vi "Set State_Measure iVIO and Resistance.vi"(0 "Semiconductor Module Context":T3, 1 "script name":string, 5 "Pins":string[](array[string])=["VDD"], 7 "Power_Pins":string[](array[string]), 9 "Published Data Ids":string[](array[string]), 11 "error in (no error)":errorcluster, 12 "SMU Settings":T2={"Level"=0.01, "Level Range"=0.1, "Limit"=1.0, "Limit Range"=6.0, "Sense"=1009} {"Sense" items=["Local"=1008, "Remote"=1009]}) -> (15 "error out":errorcluster)   [LabVIEW 2013]
uses:
  <vilib>/NI_TestStand_SemiconductorModule/NI_TestStand_Semiconductor_Module.lvlibp/PinMap/General/SemiconductorModuleContext.ctl
  <instrlib>/niDCPower/nidcpower.llb/niDCPower Sense.ctl
  <instrlib>/niHSDIO/niHSDIO.llb/niHSDIO_ctl Trigger Script - trigID Values (Ring).ctl
  <vilib>/NI_TestStand_SemiconductorModule/NI_TestStand_Semiconductor_Module.lvlibp/PinMap/DC Power/PinsToNIDCPowerSessions.vi
  <vilib>/NI_TestStand_SemiconductorModule/NI_TestStand_Semiconductor_Module.lvlibp/PinMap/General/Publish/PublishDataDouble2D.vi
  <vilib>/NI_TestStand_SemiconductorModule/NI_TestStand_Semiconductor_Module.lvlibp
panel:
  out "current measurements":dbl[][](array[numeric])
  out "R Array":dbl[][](array[numeric]) format="%#_6p"
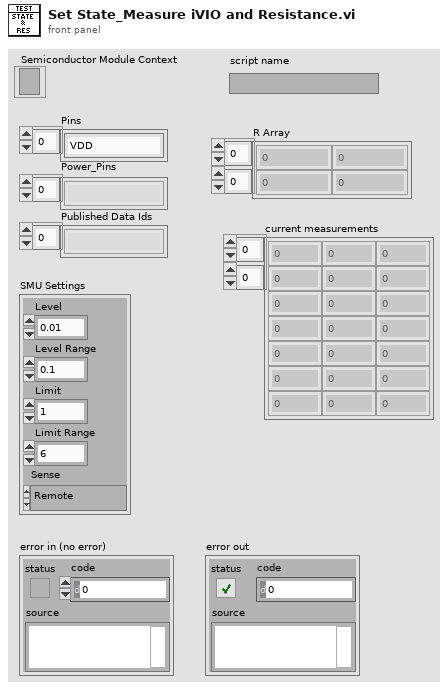
[diagram p1: front panel]
types:
  T1 = typedef "niDCPower Sense.ctl" = i32
  T2 = cluster{"Level":dbl, "Level Range":dbl, "Limit":dbl, "Limit Range":dbl, "Sense":T1}
  T3 = typedef "NI_TestStand_Semiconductor_Module.lvlibp/SemiconductorModuleContext.ctl" = refnum<k7>
  T4 = typedef "niHSDIO_ctl Trigger Script - trigID Values (Ring).ctl" = string
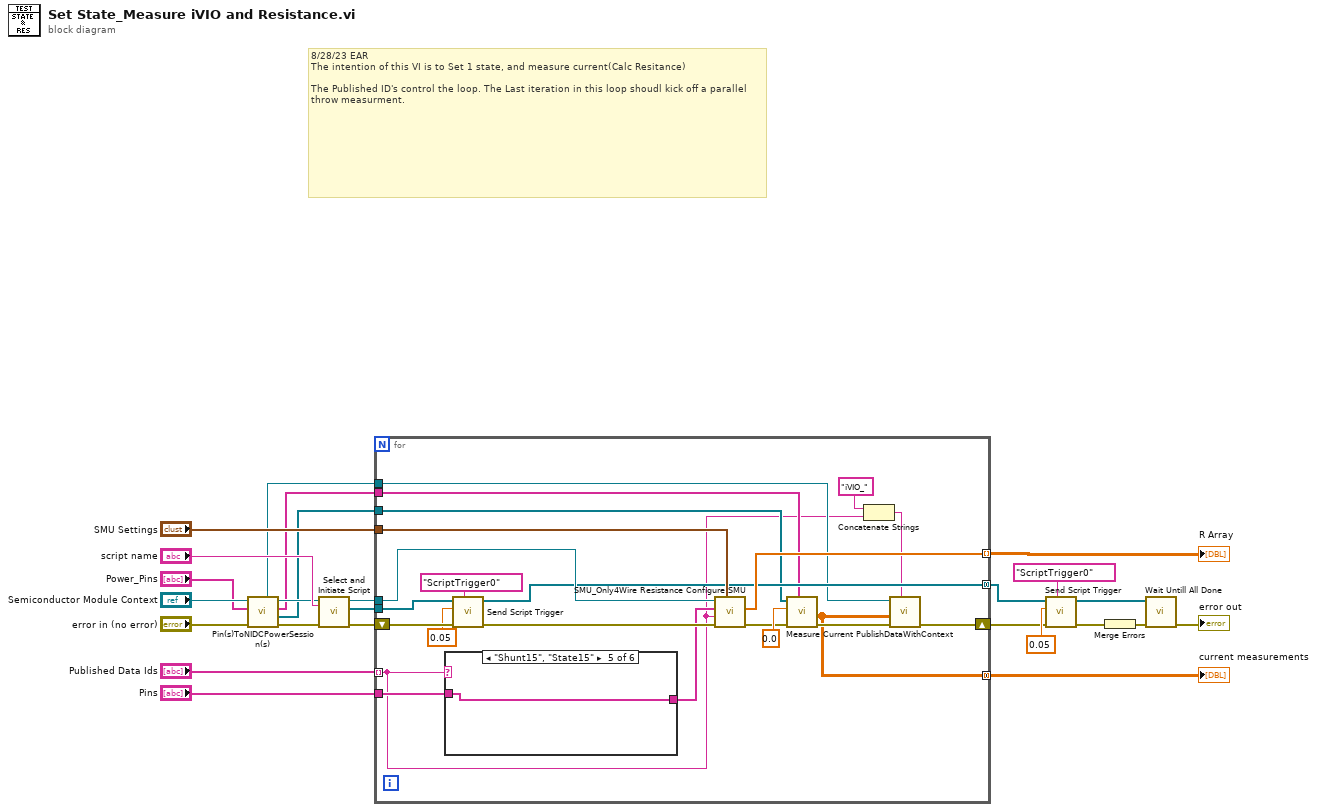
[diagram p0: block diagram]
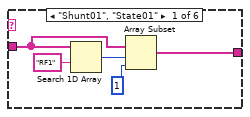
[diagram p2: hidden frame]
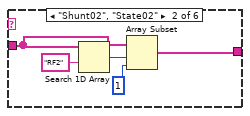
[diagram p3: hidden frame]
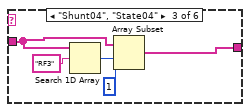
[diagram p4: hidden frame]
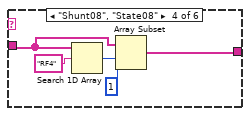
[diagram p5: hidden frame]
diagram:
  # "8/28/23 EAR\nThe intention of this VI is to Set 1 state, and measure current(Calc Resitance)\n\nThe Published ID's control the loop. The Last iteration in this loop shoudl kick off a parallel throw measurment."
  n1 = call-poly <vilib>:"Pin(s)ToNIDCPowerSession(s).vi"("error in (no error)"="error in (no error)", "Pins"="Power_Pins", "Semiconductor Module Context"="Semiconductor Module Context") -> ("error out"=w10:errorcluster, "Instrument Sessions"=w5:refnum<k15>[], "Channel Lists"=w4:string[], "Semiconductor Module Context Out"=w7:T3, "Pin Query Context"=w2:refnum<class "MultiplePinMultipleSessionQueryContext.lvclass">)  [unwired: 4 in]
  n2 = call "Select and Initiate Script.vi"("error in (no error)"=w10, "script name"="script name", "Semiconductor Module Context"=w7) -> ("error out"=w25:errorcluster, "HSDIO GEN Sessions Out"=w24:refnum<k15>[], "Semiconductor Module Context Out"=w21:T3)  [unwired: 6 in]
  n3 = for {
    tunnel: w24 -> [w46]
    tunnel: "SMU Settings" -> [w45]
    tunnel: w21 -> [w44]
    tunnel: "Published Data Ids" -> [w28] mode=indexing
    tunnel: "Pins" -> [w40]
    tunnel: [w41] -> w18 mode=indexing
    tunnel: [w38] -> w13 mode=concatenating
    shift-right: [w31] -> w3
    shift-left: w25 -> [w47]
    tunnel: w5 -> [w33]
    tunnel: w4 -> [w34]
    tunnel: w2 -> [w30]
    tunnel: [w29] -> w1 mode=concatenating
    n4 = case shown="\"Shunt15\", \"State15\"" w28 {
      tunnel: w40 -> [w51 w54 w61 w63 w68 w69]
      tunnel: [w50 w53 w60 w64 w68 w69] -> w39
      frame "Shunt01", "State01" {
        n5 = Search 1D Array(1D array=w51, element="RF1") -> (index of element=w49:i32)  [unwired: 1 in]
        n6 = Array Subset(array=w51, index=w49, length=1) -> (w50:string[])
      }
      frame "Shunt02", "State02" {
        n7 = Search 1D Array(1D array=w54, element="RF2") -> (index of element=w56:i32)  [unwired: 1 in]
        n8 = Array Subset(array=w54, index=w56, length=1) -> (w53:string[])
      }
      frame "Shunt04", "State04" {
        n9 = Search 1D Array(1D array=w61, element="RF3") -> (index of element=w59:i32)  [unwired: 1 in]
        n10 = Array Subset(array=w61, index=w59, length=1) -> (w60:string[])
      }
      frame "Shunt08", "State08" {
        n11 = Search 1D Array(1D array=w63, element="RF4") -> (index of element=w66:i32)  [unwired: 1 in]
        n12 = Array Subset(array=w63, index=w66, length=1) -> (w64:string[])
      }
      frame "Shunt15", "State15" {
      }
      frame "Shunt00", "State00", Default {
      }
    }
    n13 = call "Send Script Trigger.vi"("trigger id (script trigger 0)"=T4 "ScriptTrigger0", "error in (no error)"=w47, "Delay Time (s)"=0.05, "HSDIO Sessions In"=w46) -> ("error out"=w42:errorcluster, "HSDIO Sessions Out"=w38:refnum<k15>[])  [unwired: 6 in]
    n14 = call "SMU_Only4Wire Resistance Configure SMU.vi"("SMU Settings"=w45, "error in (no error)"=w42, "Published Data Id"=w28, "Pins"=w39, "Semiconductor Module Context"=w44) -> ("error Out"=w35:errorcluster, "R Array"=w41:dbl[])  [unwired: 4 in, 1 out]
    n15 = call "Measure Current.vi"("Channel Lists"=w34, "error in (no error)"=w35, "Delay Time (s)"=0.0, "DCPower Sessions In"=w33) -> ("error out"=w32:errorcluster, "current measurements"=w29:dbl[][])  [unwired: 5 in, 1 out]
    n16 = Concatenate Strings("iVIO_" ("Published Data Id"), w28) -> (w27:string)
    n17 = call-poly <vilib>:"PublishDataWithContext.vi"("Published Data Id"=w27, "error in (no error)"=w32, "Data In"=w29, "Pin Query Context"=w30) -> ("error out"=w31:errorcluster)  [unwired: 6 in, 1 out]
  }
  "R Array" <- w18
  "current measurements" <- w1
  n18 = call "Send Script Trigger.vi"("trigger id (script trigger 0)"=T4 "ScriptTrigger0", "error in (no error)"=w3, "Delay Time (s)"=0.05, "HSDIO Sessions In"=w13) -> ("error out"=w14:errorcluster, "HSDIO Sessions Out"=w12:refnum<k15>[])  [unwired: 6 in]
  n19 = Merge Errors(w14) -> (w17:errorcluster)
  n20 = call "Wait Untill All Done.vi"("error in (no error)"=w17, "HSDIO Sessions In"=w12) -> ("error out"=→"error out":errorcluster)  [unwired: 8 in, 1 out]
